vi "Keysight 34401a Simulator.vi"() -> ()   [LabVIEW 2021]
uses:
  <vilib>/Utility/error.llb/Error Cluster From Error Code.vi
  <vilib>/ErrorRing/Error Ring.xnode
  <vilib>/Utility/config.llb/Read Key (String).vi
  <vilib>/numeric/Random Number (Range) DBL.vi
  <vilib>/Utility/config.llb/NI_LVConfig.lvlib
panel:
  in  "Connection Timeout(wait forever: -1)":i32=500
  out "error out":errorcluster
  in  "stop":bool
  in  "Port Number":u16=50000
  in  "error in":errorcluster
  # "Keysight DMM (Agilent 34401) Simulator"
  # "How to simulate in NI MAX?\n1. Run the simulator.\n2. Open NI MAX->My System->Devices and Interfaces ->Network Devices.\n3.Right click Network Devices and Create New VISA TCP/IP Resource.\n4. Select Manual Entry of Raw Socket and click Next.\n5. Enter the Hostname as localhost and Port Number same as in this simulator.\n6. Click Validate to verify.\n7. Click Next.\n8. Enter the Alias and click Finish."
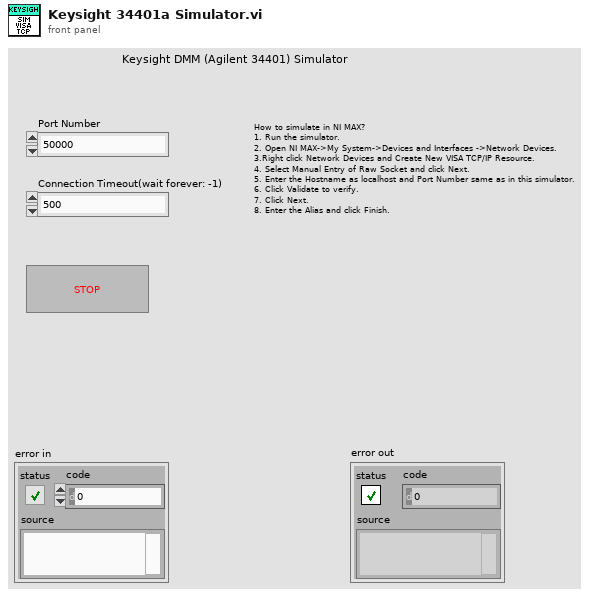
[diagram p1: front panel]
types:
  T1 = typedef "NI_LVConfig.lvlib/Config Data RefNum.ctl" = refnum<k1>
  T2 = enum16{"Standard", "Buffered", "CRLF", "Immediate"}
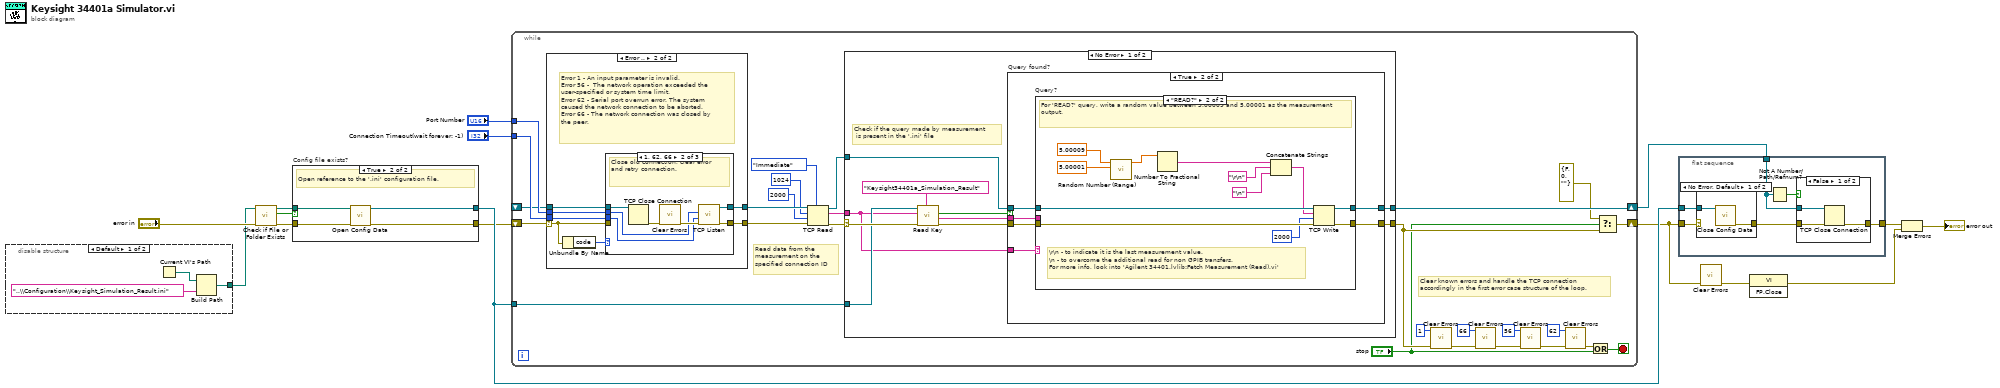
[diagram p0: block diagram]
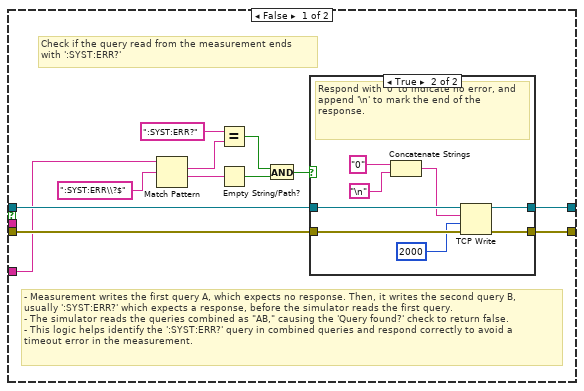
[diagram p2: hidden frame]
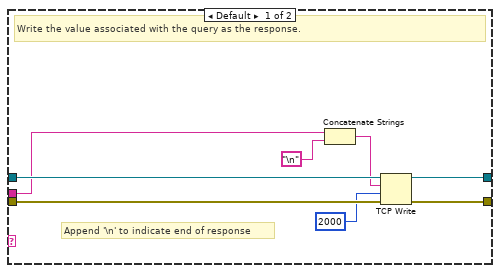
[diagram p4: hidden frame]
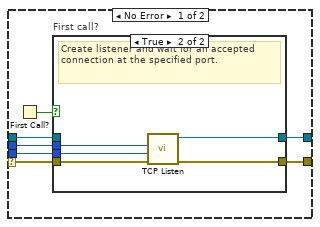
[diagram p6: hidden frame]
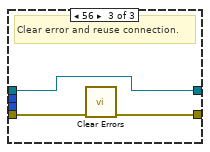
[diagram p9: hidden frame]
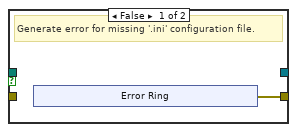
[diagram p12: hidden frame]
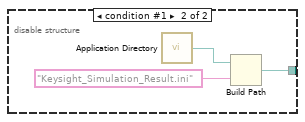
[diagram p13: hidden frame]
diagram:
  n1 = disable-structure shown="Default" {
    disable-tunnel: [w16 w21] -> w5
    frame condition #0 (active) {
      n2 = Current VI's Path() -> (path=w18:path)
      n3 = Build Path(base path=w18, name or relative path="..\\Configuration\\Keysight_Simulation_Result.ini" ("write buffer")) -> (appended path=w16:path)
    }
    frame condition #1 {
      n4 = call <vilib>:"Application Directory.vi"() -> ("Application Directory"=w19:path)
      n5 = Build Path(base path=w19, name or relative path="Keysight_Simulation_Result.ini" ("write buffer")) -> (appended path=w21:path)
    }
  }
  n6 = call <vilib>:"Check if File or Folder Exists.vi"("error in (no error)"="error in", "path"=w5) -> ("error out"=w12:errorcluster, "file or folder exists?"=w7:bool, "dup path"=w11:path)  [unwired: 7 in]
  n7 = case "Config file exists?" shown="True" w7 {
    tunnel: [_ w31] -> w15
    tunnel: w12 -> [_ w29]
    tunnel: w11 -> [_ w30]
    tunnel: [w22 w28] -> w9
    frame False {
      # "Generate error for missing '.ini' configuration file."
      n8 = xnode "Error Ring"() -> ("error out"=w22:errorcluster)
    }
    frame True {
      # "Open reference to the '.ini' configuration file."
      n9 = call <vilib>:"Open Config Data.vi"("error in (no error)"=w29, "configuration file path"=w30) -> ("error out"=w28:errorcluster, "refnum"=w31:T1)  [unwired: 7 in, 1 out]
    }
  }
  n10 = while {
    tunnel: w15 -> [w57]
    tunnel: "Port Number" -> [w52]
    tunnel: "Connection Timeout(wait forever: -1)" -> [w51]
    shift-right: [w35] -> w3
    shift-left: w9 -> [w53]
    shift-right: [w37] -> w6
    shift-left: _ -> [w46]
    stop <- w56 stop-if-true
    # "Read data from the \nmeasurement on the\nspecified connection ID"
    # "Clear known errors and handle the TCP connection\naccordingly in the first error case structure of the loop."
    n11 = case shown="Error .." w53 {
      selector: w53 -> [w125 w134]
      tunnel: [w121 w135] -> w55
      tunnel: [w120 w139] -> w54
      tunnel: w52 -> [w124 w138]
      tunnel: w51 -> [w123 w137]
      tunnel: w46 -> [w122 w136]
      frame No Error {
        n12 = First Call?() -> (First Call?: T/F=w119:bool)
        n13 = case "First call?" shown="True" w119 {
          tunnel: [w126 w132] -> w121
          tunnel: [w127 w128] -> w120
          tunnel: w125 -> [w127 w129]
          tunnel: w124 -> [_ w131]
          tunnel: w123 -> [_ w130]
          tunnel: w122 -> [w126 _]
          frame False {
            # "Pass the connection ID."
          }
          frame True {
            # "Create listener and wait for an accepted connection at the specified port."
            n14 = call <vilib>:"TCP Listen.vi"("error in (no error)"=w129, "timeout ms (wait forever: -1)"=w130, "port"=w131) -> ("error out"=w128:errorcluster, "connection ID"=w132:refnum<k5>)  [unwired: 4 in, 3 out]
          }
        }
      }
      frame Error {
        # "Error 1 - An input parameter is invalid. \nError 56 -  The network operation exceeded the \nuser-specified or system time limit. \nError 62 - Serial port overrun error. The system\ncaused the network connection to be aborted.\nError 66 - The network connection was closed by\nthe peer."
        n15 = Unbundle By Name(w134) -> ("code"=w133:i32)
        n16 = case shown="1, 62, 66" w133 {
          tunnel: [w140 w144 w150] -> w139
          tunnel: w134 -> [w140 _ w151]
          tunnel: w138 -> [_ w143 _]
          tunnel: w137 -> [_ w142 _]
          tunnel: w136 -> [w141 w148 w149]
          tunnel: [w141 w147 w149] -> w135
          frame Default {
            # "Pass connection ID."
          }
          frame 1, 62, 66 {
            # "Close old connection, clear error and retry connection."
            n17 = TCP Close Connection(connection ID=w148) -> (error out=w146:errorcluster)  [unwired: 2 in, 1 out]
            n18 = call <vilib>:"Clear Errors.vi"("error in (no error)"=w146) -> ("error out"=w145:errorcluster)  [unwired: 5 in, 1 out]
            n19 = call <vilib>:"TCP Listen.vi"("error in (no error)"=w145, "timeout ms (wait forever: -1)"=w142, "port"=w143) -> ("error out"=w144:errorcluster, "connection ID"=w147:refnum<k5>)  [unwired: 4 in, 3 out]
          }
          frame 56 {
            # "Clear error and reuse connection."
            n20 = call <vilib>:"Clear Errors.vi"("error in (no error)"=w151) -> ("error out"=w150:errorcluster)  [unwired: 5 in, 1 out]
          }
        }
      }
    }
    n21 = TCP Read(connection ID=w55, bytes to read=1024, error in (no error)=w54, 7:T2."Immediate" ("mode (standard)"), 9:2000 ("timeout ms (25000)")) -> (connection ID out=w33:refnum<k5>, data out=w58:string, error out=w38:errorcluster)
    n22 = case shown="No Error" w38 {
      selector: w38 -> [w68 w118]
      tunnel: w58 -> [w60 _]
      tunnel: w57 -> [w67 _]
      tunnel: [w64 w118] -> w36
      tunnel: [w66 w117] -> w37
      tunnel: w33 -> [w59 w117]
      frame No Error {
        # "Check if the query made by measurement\n is present in the '.ini' file"
        n23 = call-poly <vilib>:"Read Key.vi"("section"="Keysight34401a_Simulation_Result", "error in (no error)"=w68, "key"=w60, "refnum"=w67) -> ("error out"=w65:errorcluster, "value"=w61:string, "found?"=w63:bool)  [unwired: 4 in, 1 out]
        n24 = case "Query found?" shown="True" w63 {
          tunnel: w65 -> [w80 w96]
          tunnel: [w79 w95] -> w64
          tunnel: w59 -> [w78 w94]
          tunnel: [w77 w93] -> w66
          tunnel: w61 -> [_ w92]
          tunnel: w60 -> [w71 w91]
          frame False {
            # "- Measurement writes the first query A, which expects no response. Then, it writes the second query B,\nusually ':SYST:ERR?' which expects a response, before the simulator reads the first query.\n- The simulator reads the queries combined as \"AB,\" causing the 'Query found?' check to return false.\n- This logic helps identify the ':SYST:ERR?' query in combined queries and respond correctly to avoid a\ntimeout error in the measurement."
            # "Check if the query read from the measurement ends\nwith ':SYST:ERR?'"
            n25 = Match Pattern(string=w71, regular expression=":SYST:ERR\\?$") -> (match substring=w74:string, after substring=w75:string)  [unwired: 1 in, 2 out]
            n26 = Equal?(x=":SYST:ERR?" ("y"), y=w74) -> (x = y?=w69:bool)
            n27 = Empty String/Path?(string/path=w75) -> (empty?=w70:bool)
            n28 = And(x=w69, y=w70) -> (x .and. y?=w72:bool)
            n29 = case "Query ends with ':SYST:ERR?' ?" shown="True" w72 {
              tunnel: w80 -> [w82 w87]
              tunnel: [w82 w88] -> w79
              tunnel: w78 -> [w81 w90]
              tunnel: [w81 w89] -> w77
              frame False {
                # "Pass"
              }
              frame True {
                # "Respond with '0' to indicate no error, and append '\\n' to mark the end of the response."
                n30 = Concatenate Strings("0" ("string"), "\n") -> (w83:string)
                n31 = TCP Write(connection ID=w90, data in=w83, error in (no error)=w87, 9:2000 ("timeout ms (25000)")) -> (connection ID out=w89:refnum<k5>, error out=w88:errorcluster)  [unwired: 1 out]
              }
            }
          }
          frame True {
            n32 = case "Query?" shown="\"READ?\"" w91 {
              tunnel: w96 -> [w104 w116]
              tunnel: [w103 w115] -> w95
              tunnel: w94 -> [w102 w114]
              tunnel: [w101 w110] -> w93
              tunnel: w92 -> [w97 _]
              frame Default {
                # "Append '\\n' to indicate end of response"
                # "Write the value associated with the query as the response."
                n33 = Concatenate Strings(w97, "\n") -> (w98:string)
                n34 = TCP Write(connection ID=w102, data in=w98, error in (no error)=w104, 9:2000 ("timeout ms (25000)")) -> (connection ID out=w101:refnum<k5>, error out=w103:errorcluster)  [unwired: 1 out]
              }
              frame "READ?" {
                # "\\r\\n - to indicate it is the last measurement value.\n\\n - to overcome the additional read for non GPIB transfers.\nFor more info, look into 'Agilent 34401.lvlib:Fetch Measurement (Read).vi'"
                # "For 'READ?' query, write a random value between 5.00009 and 5.00001 as the measurement output."
                n35 = call-poly <vilib>:"Random Number (Range).vi"("lower bound (0)"=5.00001, "upper bound (100)"=5.00009) -> ("number"=w109:dbl)  [unwired: 9 in]
                n36 = Number To Fractional String(number=w109) -> (F-format string=w105:string)  [unwired: 3 in]
                n37 = Concatenate Strings(w105, "\r\n", "\n") -> (w106:string)
                n38 = TCP Write(connection ID=w114, data in=w106, error in (no error)=w116, 9:2000 ("timeout ms (25000)")) -> (connection ID out=w110:refnum<k5>, error out=w115:errorcluster)  [unwired: 1 out]
              }
            }
          }
        }
      }
      frame Error {
      }
    }
    n39 = call <vilib>:"Clear Errors.vi"("error in (no error)"=w36, "specific error code to clear (0: all)"=1) -> ("error out"=w45:errorcluster)  [unwired: 4 in, 1 out]
    n40 = call <vilib>:"Clear Errors.vi"("error in (no error)"=w45, "specific error code to clear (0: all)"=66) -> ("error out"=w48:errorcluster)  [unwired: 4 in, 1 out]
    n41 = call <vilib>:"Clear Errors.vi"("error in (no error)"=w48, "specific error code to clear (0: all)"=56) -> ("error out"=w50:errorcluster)  [unwired: 4 in, 1 out]
    n42 = call <vilib>:"Clear Errors.vi"("error in (no error)"=w50, "specific error code to clear (0: all)"=62) -> ("error out"=w43:errorcluster)  [unwired: 4 in, 1 out]
    n43 = Or(x=w43, y="stop") -> (x .or. y?=w56:bool)
    n44 = Select(t=errorcluster {"status"=FALSE, "code"=0, "source"=""}, s="stop", f=w36) -> (s? t:f=w35:errorcluster)
  }
  n45 = flat-sequence {
    tunnel: w15 -> [w157]
    tunnel: [w155] -> w14
    tunnel: w6 -> [w154]
    tunnel: w3 -> [w152]
    frame #0 {
      n46 = case shown="No Error, Default" w152 {
        selector: w152 -> [_ w160]
        tunnel: w157 -> [w159 _]
        tunnel: [w158 w160] -> w156
        frame No Error {
          n47 = call <vilib>:"Close Config Data.vi"("refnum"=w159) -> ("error out"=w158:errorcluster)  [unwired: 9 in, 1 out]
        }
        frame Error {
        }
      }
      n48 = Not A Number/Path/Refnum?(number/path/refnum=w154) -> (NaN/Path/Refnum?=w153:bool)
      n49 = case shown="False" w153 {
        tunnel: w156 -> [w163 w164]
        tunnel: [w162 w164] -> w155
        tunnel: w154 -> [w161 _]
        frame False {
          n50 = TCP Close Connection(connection ID=w161, error in (no error)=w163) -> (error out=w162:errorcluster)  [unwired: 1 in, 1 out]
        }
        frame True {
        }
      }
    }
  }
  n51 = call <vilib>:"Clear Errors.vi"("error in (no error)"=w3) -> ("error out"=w4:errorcluster)  [unwired: 5 in, 1 out]
  n52 = invoke class="VI" method="FP.Close"(error in=w4) -> (error out=w2:errorcluster)  [unwired: 2 in, 2 out]
  n53 = Merge Errors(w14, w2) -> (→"error out":errorcluster)
